vi "Keithley 2400 Voltage Set.vi"(8 "error in (no error)":errorcluster, 10 "Voltage Level":dbl, 11 "VISA Refnum in":refnum<visa-resource-name>) -> (0 "error out":errorcluster, 3 "VISA Refnum out":refnum<visa-resource-name>)   [LabVIEW 2019]
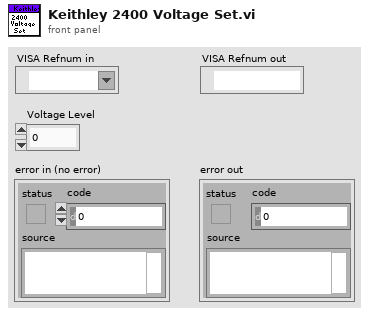
[diagram p1: front panel]
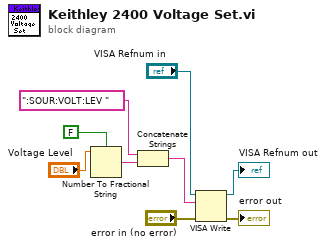
[diagram p0: block diagram]
diagram:
  n1 = Number To Fractional String(use system decimal point (T)=FALSE, number="Voltage Level") -> (F-format string=w2:string)  [unwired: 2 in]
  n2 = Concatenate Strings(":SOUR:VOLT:LEV ", w2) -> (w4:string)
  n3 = VISA Write(VISA resource name="VISA Refnum in", write buffer=w4, error in (no error)="error in (no error)") -> (VISA resource name out=→"VISA Refnum out":refnum<visa-resource-name>, error out=→"error out":errorcluster)  [unwired: 1 out]
